vi "Close DB.vi"(8 "error in":errorcluster, 11 "LV-ORM in":refnum<class "LV-ORM.lvclass">) -> (0 "error out":errorcluster, 3 "LV-ORM out":refnum<class "LV-ORM.lvclass">)   [LabVIEW 2018, in "LV-ORM.lvclass"]
uses:
  LV-ORM.lvclass
  <vilib>/addons/database/Connection.llb/Conn ObjectReference.ctl
  LV-ORM.lvclass/LV-ORM.ctl
  <vilib>/addons/database/NI_Database_API.lvlib
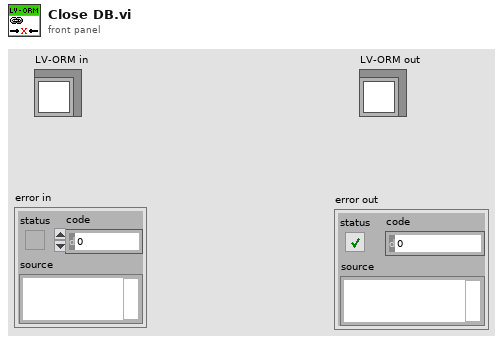
[diagram p1: front panel]
types:
  T1 = typedef "NI_Database_API.lvlib/Conn ObjectReference.ctl" = refnum<k1>
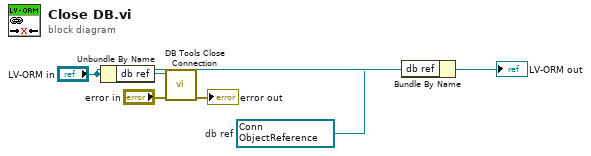
[diagram p0: block diagram]
diagram:
  w1 = T1 refnum items=["Connection"]  # db ref
  n1 = Unbundle By Name("LV-ORM in") -> ("db ref"=w4:T1)
  n2 = call <vilib>:"DB Tools Close Connection.vi"("error in (no error)"="error in", "connection reference"=w4) -> ("error out"=→"error out":errorcluster)  [unwired: 5 in]
  n3 = Bundle By Name(cluster="LV-ORM in", "db ref"=w1) -> (→"LV-ORM out":refnum<class "LV-ORM.lvclass">)
